vi "DDS Close.vi"(8 "error in (no error)":errorcluster, 11 "DDS ref in":T1={"NI USB-8451 device reference"="", "DIO port"=0, "Serial Clock Rate [kHz]"=1000}) -> (0 "error out":errorcluster)   [LabVIEW 2013, in "DDS.lvlib"]
doc: "Disables the SPI interface and sets the TTL lines to a high-impedance state then closes the USB-8451 device reference."
uses:
  DDS.lvlib
  Controls/DDS Box Device Reference.ctl
  <vilib>/ni845x/ni845x.llb/ni845xControl.ctl
  <vilib>/ni845x/ni845x.llb/NI-845x Close Device Reference.vi
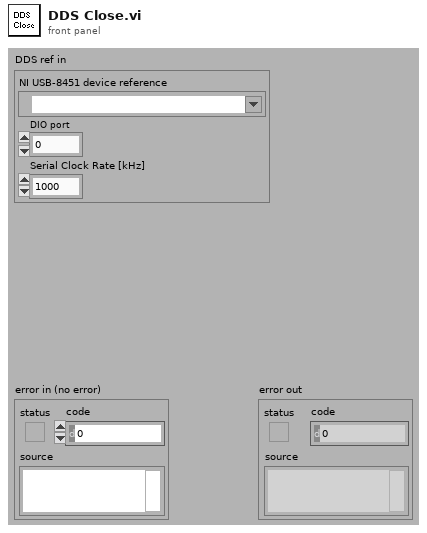
[diagram p1: front panel]
types:
  T1 = typedef "DDS.lvlib/DDS Box Device Reference.ctl" = cluster{"NI USB-8451 device reference":T2, "DIO port":u8, "Serial Clock Rate [kHz]":u16}
  T2 = typedef "ni845xControl.ctl" = refnum<k21>
  T3 = typedef "ni845xSpiScriptControl.ctl" = refnum<k20>
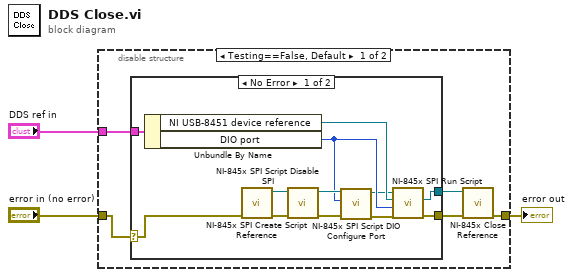
[diagram p0: block diagram]
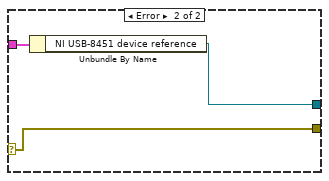
[diagram p2: hidden frame]
diagram:
  n1 = disable-structure shown="Testing==False, Default" {
    disable-tunnel: "DDS ref in" -> [w6 _]
    disable-tunnel: [w5 w24] -> w2
    disable-tunnel: "error in (no error)" -> [w4 w24]
    frame condition #0 (active) {
      n2 = case shown="No Error" w4 {
        selector: w4 -> [w9 w21]
        tunnel: [w18 w21] -> w8
        tunnel: [w17 w22] -> w7
        tunnel: w6 -> [w16 w23]
        frame No Error {
          n3 = Unbundle By Name(w16) -> ("NI USB-8451 device reference"=w15:T2, "DIO port"=w12:u8)
          n4 = call <vilib>:"NI-845x SPI Create Script Reference.vi"("error in (no error)"=w9) -> ("error out"=w20:errorcluster, "spi script reference"=w19:T3)  [unwired: 9 in]
          n5 = call <vilib>:"NI-845x SPI Script Disable SPI.vi"("error in (no error)"=w20, "spi script reference in"=w19) -> ("error out"=w14:errorcluster, "spi script reference out"=w13:T3)  [unwired: 8 in]
          n6 = call <vilib>:"NI-845x SPI Script DIO Configure Port.vi"("error in (no error)"=w14, "port number (0)"=w12, "spi script reference in"=w13) -> ("error out"=w11:errorcluster, "spi script reference out"=w10:T3)  [unwired: 7 in]
          n7 = call <vilib>:"NI-845x SPI Run Script.vi"("error in (no error)"=w11, "port (0)"=w12, "device reference in"=w15, "spi script reference in"=w10) -> ("error out"=w18:errorcluster, "device reference out"=w17:T2)  [unwired: 5 in, 1 out]
        }
        frame Error {
          n8 = Unbundle By Name(w23) -> ("NI USB-8451 device reference"=w22:T2)
        }
      }
      n9 = call-poly <vilib>:"NI-845x Close Reference.vi"("error in (no error)"=w8, "device reference"=w7) -> ("error out"=w5:errorcluster)  [unwired: 9 in]
    }
    frame condition #1 {
    }
  }
  "error out" <- w2
